vi "GEA2 Write ERD.vi"(0 "GEA2 Reference In":refnum<k24>, 1 "Retry Count":i32=5, 2 "Read Timeout (ms)":u32=500, 5 "GEA Inputs":T1 {"Destination" format="%.0x"; "Source" format="%.0x"}, 7 "Write ERD List":T2[](array[typedef]) {"ERD Number" format="%.0x"}, 11 "Error In":errorcluster, 13 "Verify ERD Response?":bool=TRUE) -> (4 "GEA2 Reference Out":refnum<k24>, 6 "Raw Data Out":string, 15 "Error Out":errorcluster)   [LabVIEW 2014, in "GEA2_Toolkit.lvlib"]
doc: "This VI writes an array of ERDs with a single command. The data type is used to convert the Data from the type specified to a hexidecimal string before sending it."
uses:
  library/GEA2_Toolkit.lvlib
  C:/Automation/DLLs/PC Tools .NET/GeaCommunication.dll
  Automation/DLLs/PC Tools .NET/GeaCommunication.dll
  type defs/ERD Write Data In.ctl
  type defs/Source_Destination.ctl
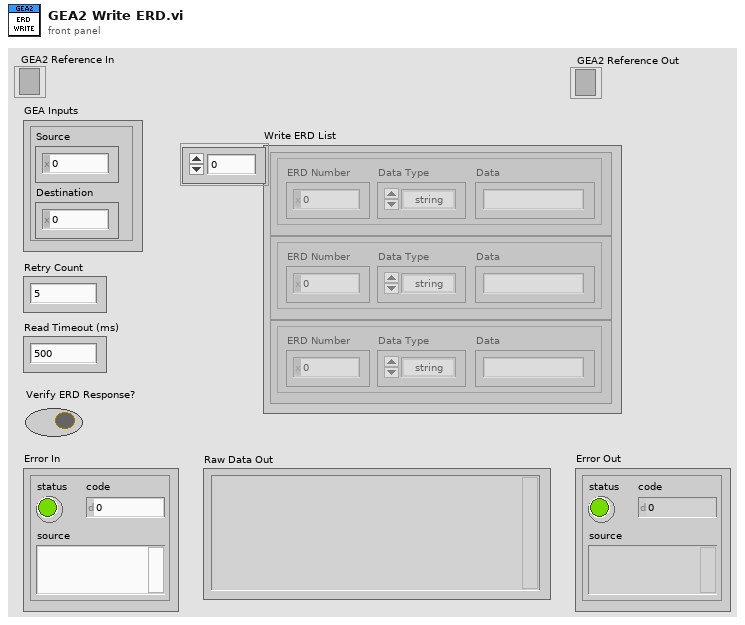
[diagram p1: front panel]
types:
  T1 = typedef "GEA2_Toolkit.lvlib/Source_Destination.ctl" = cluster{"Source":u8, "Destination":u8}
  T2 = typedef "GEA2_Toolkit.lvlib/ERD Write Data In.ctl" = cluster{"ERD Number":u16, "Data Type":enum16{"string", "boolean", "uint8_t", "uint16_t", "uint32_t"}, "Data":string}
  T3 = typedef "GEA2_Toolkit.lvlib/Data In.ctl" = cluster{"Source":u8, "Destination":u8, "Command":u8, "Message":string}
  T4 = typedef "GEA2_Toolkit.lvlib/Data Out.ctl" = cluster{"Source":u8, "Destination":u8, "Command":u8, "Length":u8, "CRC":u16, "Message":string}
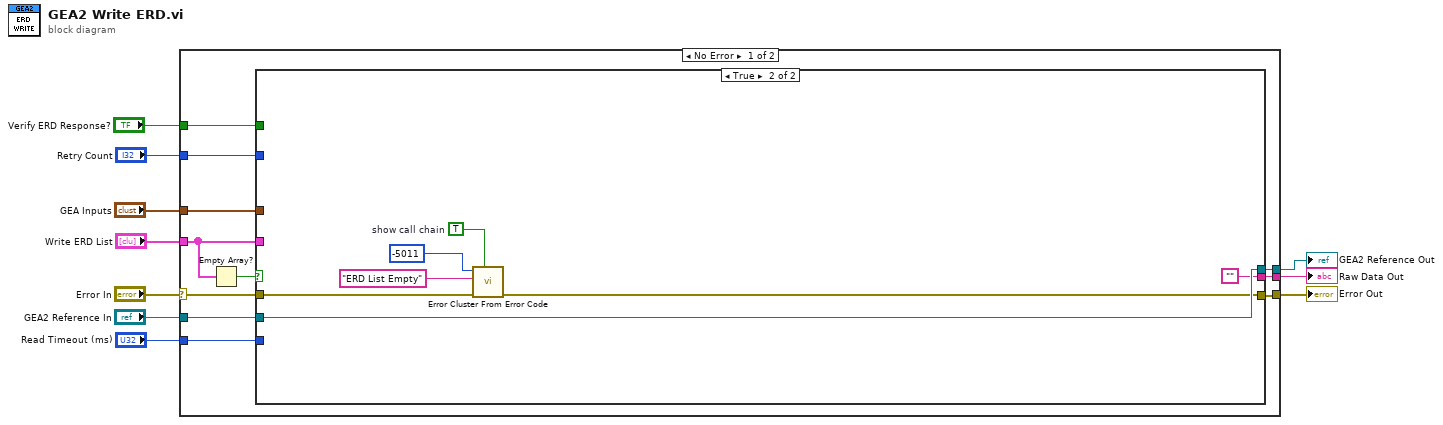
[diagram p0: block diagram]
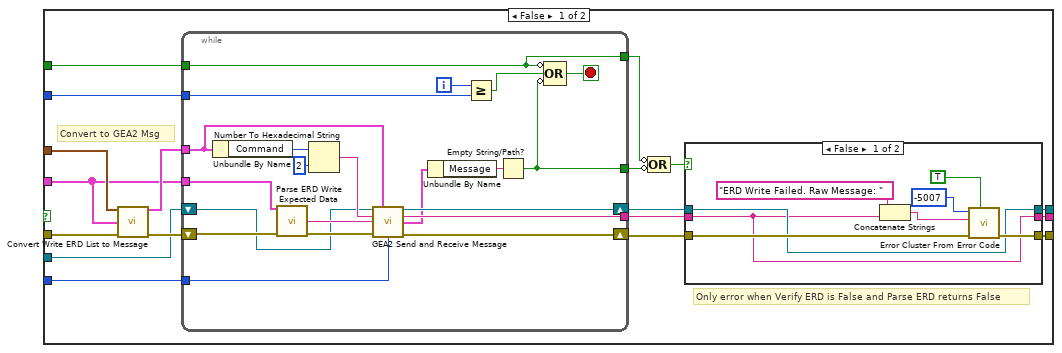
[diagram p2: hidden frame]
diagram:
  n1 = case shown="No Error" "Error In" {
    selector: "Error In" -> [w14 w79]
    tunnel: "GEA2 Reference In" -> [w13 w80]
    tunnel: "Write ERD List" -> [w12 _]
    tunnel: "Verify ERD Response?" -> [w21 _]
    tunnel: "GEA Inputs" -> [w15 _]
    tunnel: [w17 _] -> w5
    tunnel: [w18 w79] -> w4
    tunnel: "Read Timeout (ms)" -> [w20 _]
    tunnel: "Retry Count" -> [w19 _]
    tunnel: [w16 w80] -> w1
    frame No Error {
      n2 = Empty Array?(array=w12) -> (empty?=w11:bool)
      n3 = case shown="True" w11 {
        tunnel: w21 -> [w39 _]
        tunnel: w20 -> [w38 _]
        tunnel: w19 -> [w37 _]
        tunnel: [w35 w73] -> w18
        tunnel: [w34 ""] -> w17
        tunnel: [w31 w78] -> w16
        tunnel: w15 -> [w27 _]
        tunnel: w14 -> [w26 w77]
        tunnel: w13 -> [w24 w78]
        tunnel: w12 -> [w22 _]
        frame False {
          # "Only error when Verify ERD is False and Parse ERD returns False"
          # "Convert to GEA2 Msg"
          n4 = call "Convert Write ERD List to Message.vi"("GEA Inputs"=w27, "Write ERD List"=w22, "Error In"=w26) -> ("GEA Message"=w23:T3, "Error Out"=w25:errorcluster)  [unwired: 11 in]
          n5 = while {
            tunnel: w23 -> [w62]
            tunnel: [w71] -> w33
            tunnel: w39 -> [w63]
            tunnel: w38 -> [w69]
            tunnel: w37 -> [w67]
            tunnel: [w56] -> w29
            tunnel: [w63] -> w30
            tunnel: w22 -> [w53]
            shift-right: [w70] -> w36
            shift-left: w25 -> [w55]
            shift-right: [w64] -> w32
            shift-left: w24 -> [w51]
            i -> [w68]
            stop <- w65 stop-if-true
            n6 = Unbundle By Name(w62) -> ("Command"=w61:u8)
            n7 = call "Parse ERD Write Expected Data.vi"("Write ERD List"=w53, "Error In"=w55) -> ("Expected Data"=w52:string, "Error Out"=w54:errorcluster)  [unwired: 12 in]
            n8 = Number To Hexadecimal String(1:i16 2 ("width (-)"), 2:w61) -> (0:w59:string)
            n9 = call "GEA2 Send and Receive Message.vi"("GEA2 Reference In"=w51, "Input Data"=w62, "Read Timeout (ms)"=w69, "Expected Command"=w59, "Expected Data"=w52, "Error In"=w54) -> ("GEA2 Reference Out"=w64:refnum<k24>, "Raw Data Out"=w71:string, "Converted Data Out"=w58:T4, "Error Out"=w70:errorcluster)  [unwired: 6 in]
            n10 = Unbundle By Name(w58) -> ("Message"=w57:string)
            n11 = Greater Or Equal?(x=w68, y=w67) -> (x >= y?=w66:bool)
            n12 = Empty String/Path?(string/path=w57) -> (empty?=w56:bool)
            n13 = Compound Arithmetic op=OR(invert w63, w66, invert w56) -> (w65:bool)
          }
          n14 = Compound Arithmetic op=OR(invert w30, invert w29) -> (w28:bool)
          n15 = case shown="False" w28 {
            tunnel: w36 -> [w47 w50]
            tunnel: [w46 w50] -> w35
            tunnel: [w40 w49] -> w34
            tunnel: w33 -> [w40 w49]
            tunnel: w32 -> [w43 w48]
            tunnel: [w43 w48] -> w31
            frame False {
              n16 = Concatenate Strings("ERD Write Failed. Raw Message: " ("error message (\"\")"), w40) -> (w41:string)
              n17 = call <vilib>:"Error Cluster From Error Code.vi"("show call chain? (False)"=TRUE, "error in (no error)"=w47, "error message (\"\")"=w41, "error code (0)"=-5007) -> ("error out"=w46:errorcluster)  [unwired: 5 in]
            }
            frame True {
            }
          }
        }
        frame True {
          w74 = TRUE  # show call chain
          n18 = call <vilib>:"Error Cluster From Error Code.vi"("show call chain? (False)"=w74, "error in (no error)"=w77, "error message (\"\")"="ERD List Empty" ("error message (\"\")"), "error code (0)"=-5011) -> ("error out"=w73:errorcluster)  [unwired: 5 in]
        }
      }
    }
    frame Error {
    }
  }
  "Raw Data Out" <- w5
  "Error Out" <- w4
  "GEA2 Reference Out" <- w1
